vi "Сканер.vi"() -> ()   [LabVIEW 2016]
uses:
  <vilib>/Instr/_visa.llb/VISA Open Access Mode.ctl
  <vilib>/Instr/_visa.llb/VISA Configure Serial Port (Instr).vi
panel:
  out "duplicate session (F)":bool
  out "read buffer":string
  out "Gauge":dbl(knob)
  out "ScrollPosBool":bool
  out "Serial Settings:Number of Bytes at Serial Port":u32
  in  "XON/XOFF Символ":cluster{"XON":u8, "XOFF":u8}={"XON"=17, "XOFF"=19} {"XOFF" items=["NUL", "SOH", "STX", "ETX", "EOT", "ENQ", "ACK", "BEL", "BS", "HT", "LF", "VT", "FF", "CR", "SO", "SI", "DLE", "DC1", "DC2", "DC3", "DC4", "NAK", "SYN", "ETB", "CAN", "EM", "SUB", "ESC", "FS", "GS", "RS", "US", "SP", "!", "\"", "#", "$", "%", "&", "'", "(", ")", "*", "+", ",", "- (-)", ".", "/", "0", "1", "2", "3", "4", "5", "6", "7", "8", "9", ":", ";", "<", "=", ">", "?", "@", "A", "B", "C", "D", "E", "F", "G", "H", "I", "J", "K", "L", "M", "N", "O", "P", "Q", "R", "S", "T", "U", "V", "W", "X", "Y", "Z", "[", "\\", "]", "^", "_", "`", "a", "b", "c", "d", "e", "f", "g", "h", "i", "j", "k", "l", "m", "n", "o", "p", "q", "r", "s", "t", "u", "v", "w", "x", "y", "z", "{", "|", "}", "~"]; "XON" items=["NUL", "SOH", "STX", "ETX", "EOT", "ENQ", "ACK", "BEL", "BS", "HT", "LF", "VT", "FF", "CR", "SO", "SI", "DLE", "DC1", "DC2", "DC3", "DC4", "NAK", "SYN", "ETB", "CAN", "EM", "SUB", "ESC", "FS", "GS", "RS", "US", "SP", "!", "\"", "#", "$", "%", "&", "'", "(", ")", "*", "+", ",", "- (-)", ".", "/", "0", "1", "2", "3", "4", "5", "6", "7", "8", "9", ":", ";", "<", "=", ">", "?", "@", "A", "B", "C", "D", "E", "F", "G", "H", "I", "J", "K", "L", "M", "N", "O", "P", "Q", "R", "S", "T", "U", "V", "W", "X", "Y", "Z", "[", "\\", "]", "^", "_", "`", "a", "b", "c", "d", "e", "f", "g", "h", "i", "j", "k", "l", "m", "n", "o", "p", "q", "r", "s", "t", "u", "v", "w", "x", "y", "z", "{", "|", "}", "~"]}
  in  "Ошибка порта":T1
  in  "Номер COM порта":refnum<visa-resource-name>
  in  "Clear":bool
  in  "ReadStringON":bool
  in  "WriteStringON":bool
  in  "В конце записи добавить идентификатор завершения":bool=TRUE
  out "IndStartStop":bool
  in  "Exit":bool
  in  "Start":bool
  in  "Stop":bool
  out "Return Count Read":u32
  in  "В конце чтения добавить идентификатор завершения":bool=TRUE
  in  "Идентификатор завершения":u8=10 format="%.0x"
  out "Read String":string
  out "Return Count Write":u32
  in  "Write String":string="*IDN?"
  in  "Параметры порта":T2={"Бит в секунду: "=9600, "Биты данных:"=8, "Чётность"=0, "Стоповые биты"=10, "Управление потоком"=0} {"Управление потоком" items=["Нет"=0, "Xon/Xoff"=1, "RTS/CTS"=2, "DTR/DSR"=4]; "Стоповые биты" items=["1.0"=10, "1.5"=15, "2.0"=20]; "Чётность" items=["Нет", "Нечётный", "Чётный", "Маркер", "Пробел"]; "Биты данных:" items=["4"=4, "5"=5, "6"=6, "7"=7, "8"=8]; "Бит в секунду:" items=["75"=75, "110"=110, "134"=134, "150"=150, "300"=300, "600"=600, "1200"=1200, "1800"=1800, "2400"=2400, "4800"=4800, "7200"=7200, "9600"=9600, "14400"=14400, "19200"=19200, "28800"=28800, "38400"=38400, "56000"=56000, "57600"=57600, "115200"=115200, "128000"=128000, "230400"=230400]}
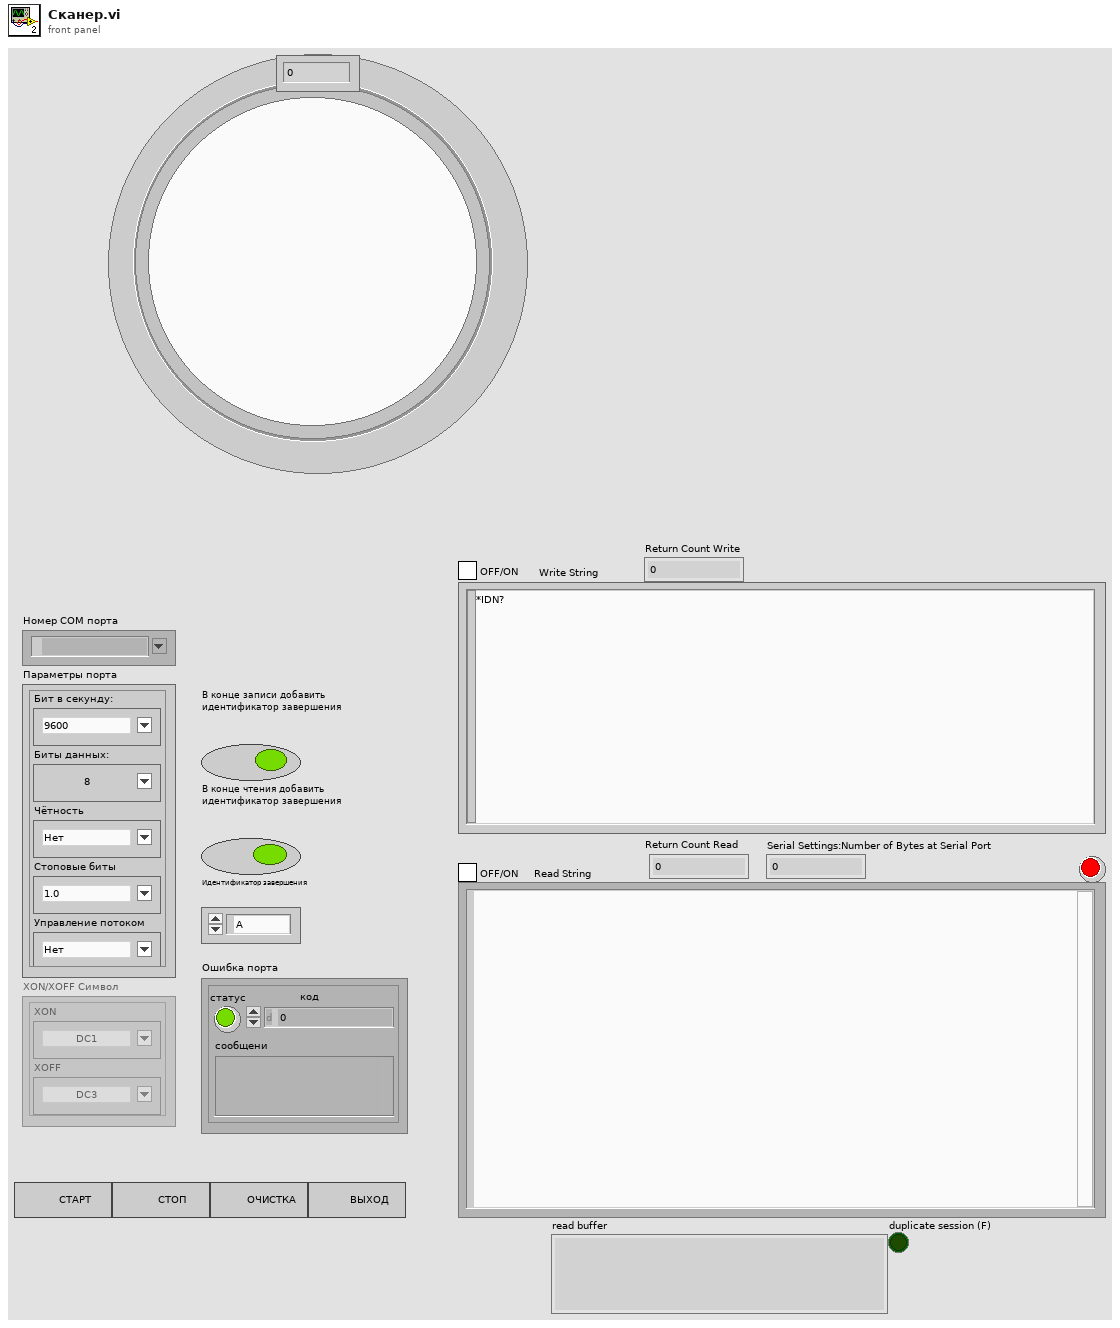
[diagram p1: front panel]
types:
  T1 = cluster{"статус":bool, "код":i32, "сообщени":string}
  T2 = cluster{"Бит в секунду: ":u32, "Биты данных:":u16, "Чётность":u16, "Стоповые биты":u16, "Управление потоком":u16}
  T3 = enum8{"Enabled", "Disabled", "Disabled and Grayed Out"}
  T4 = typedef "VISA Open Access Mode.ctl" = u32
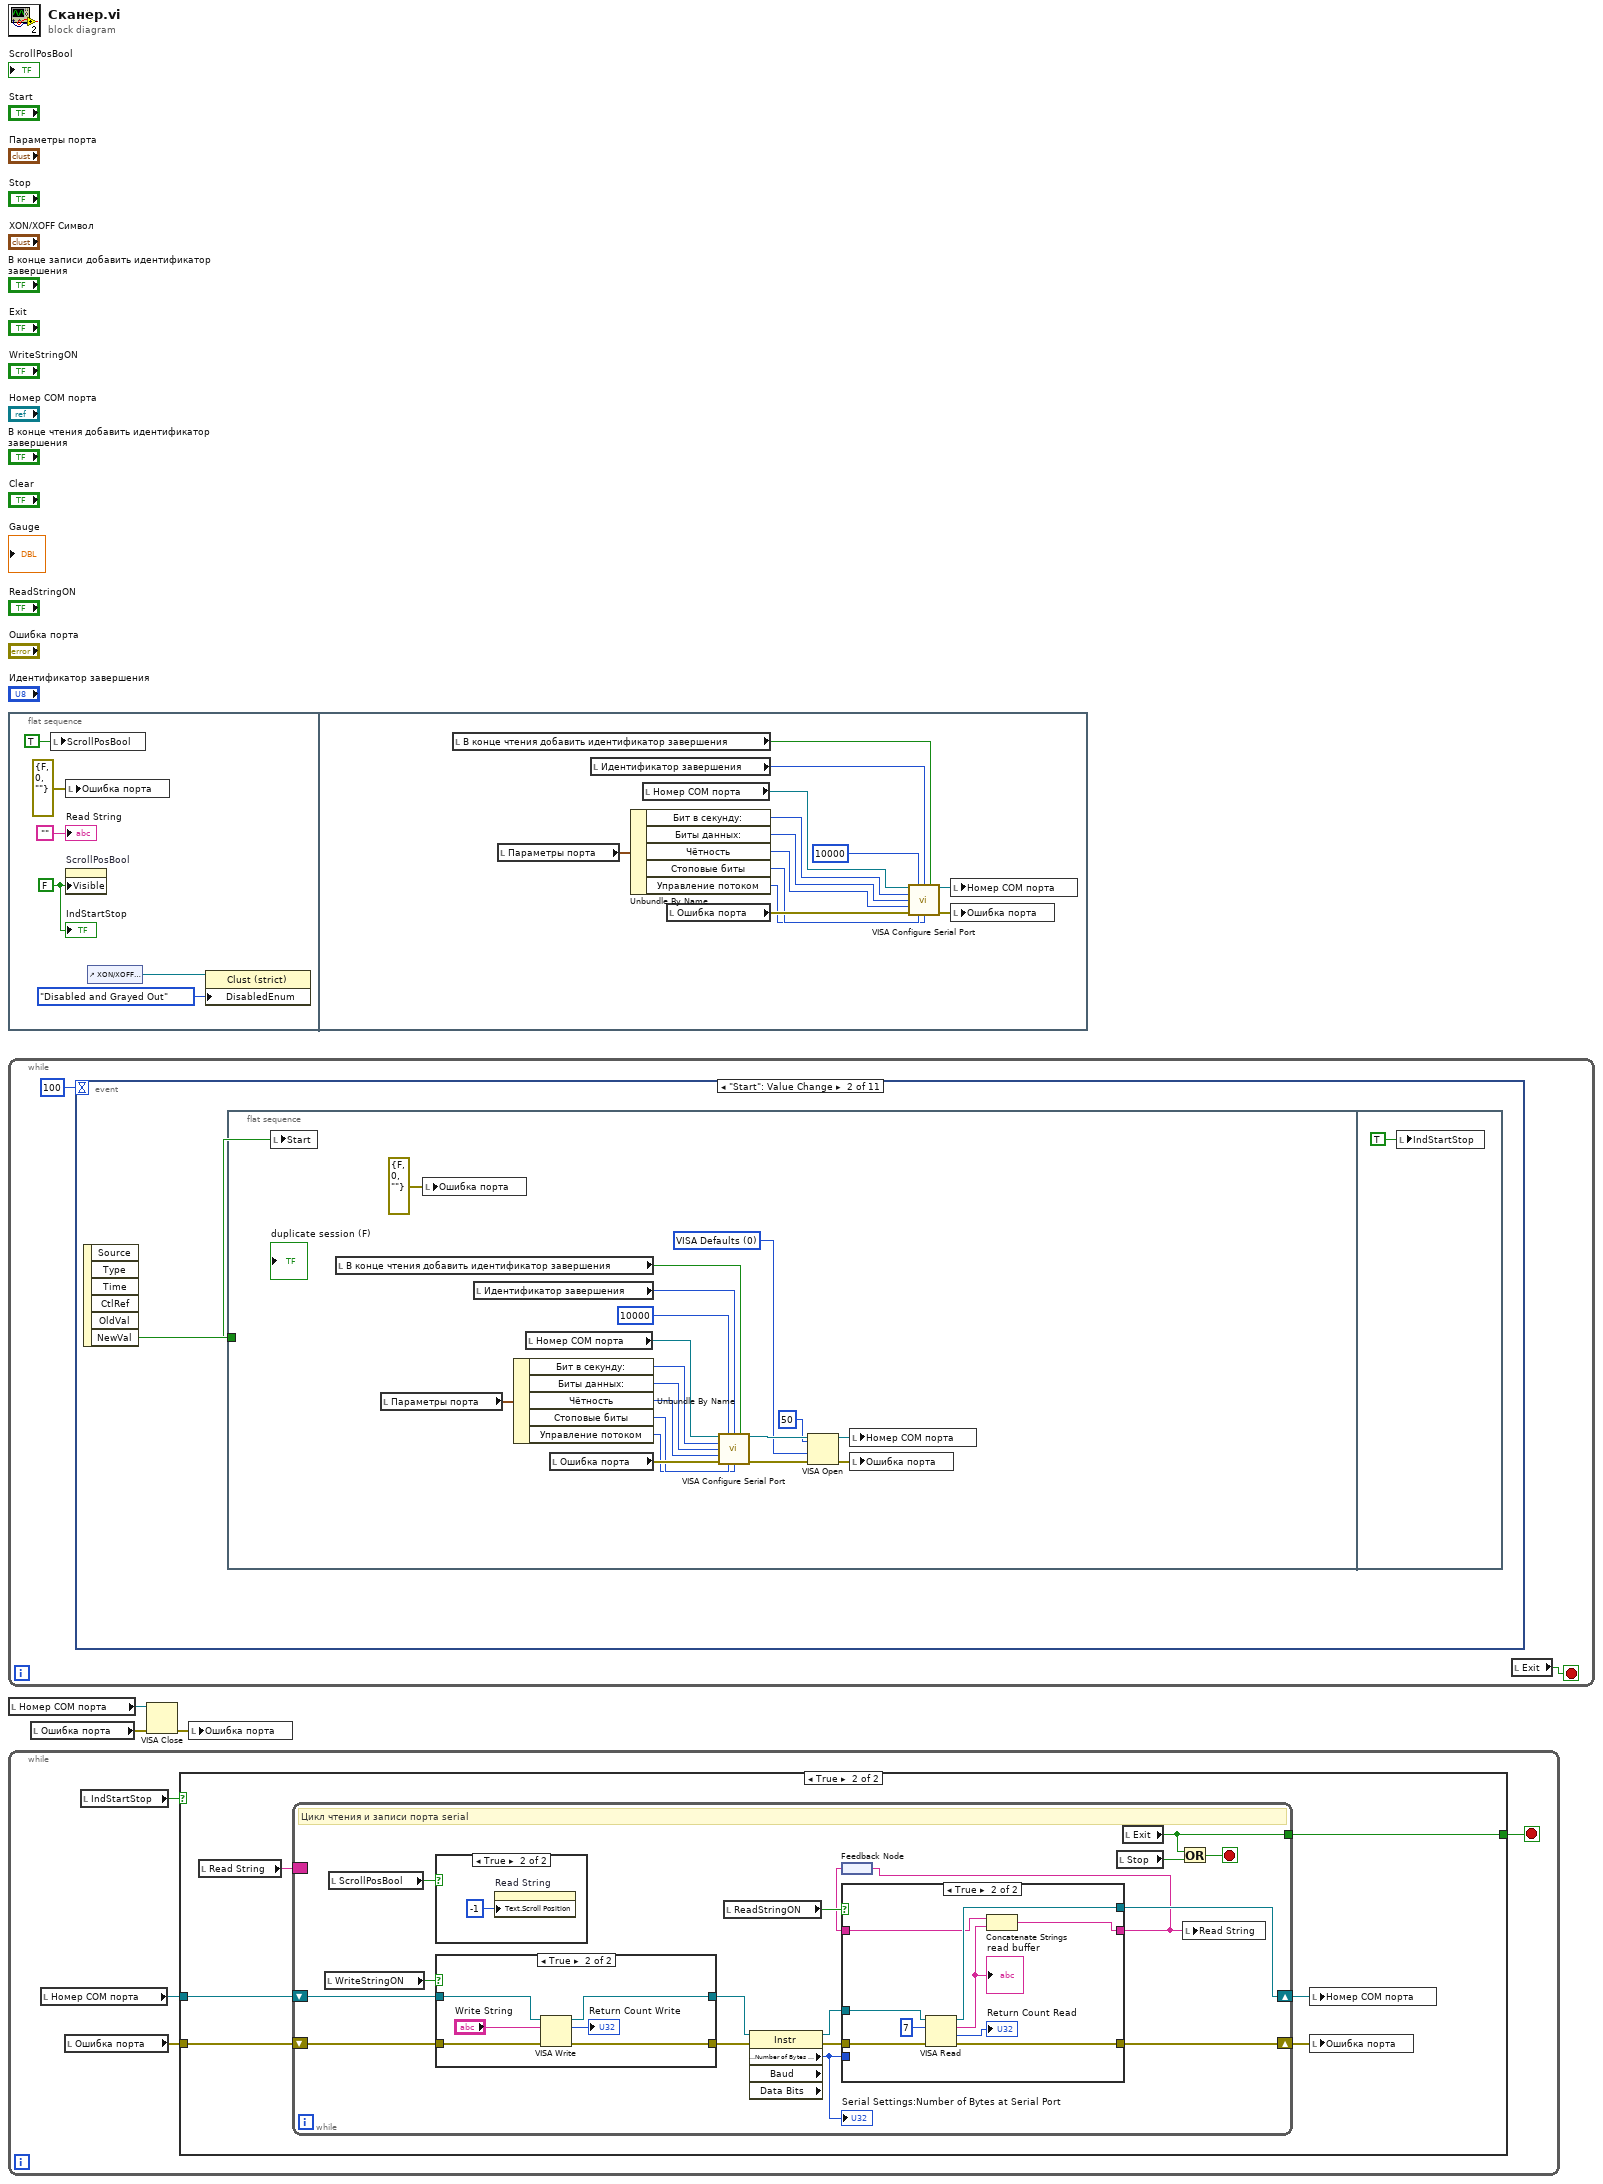
[diagram p0: block diagram]
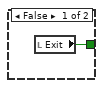
[diagram p2: hidden frame]
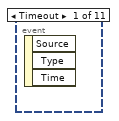
[diagram p6: hidden frame]
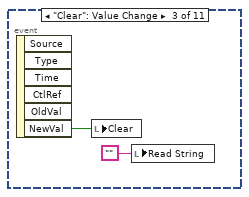
[diagram p7: hidden frame]
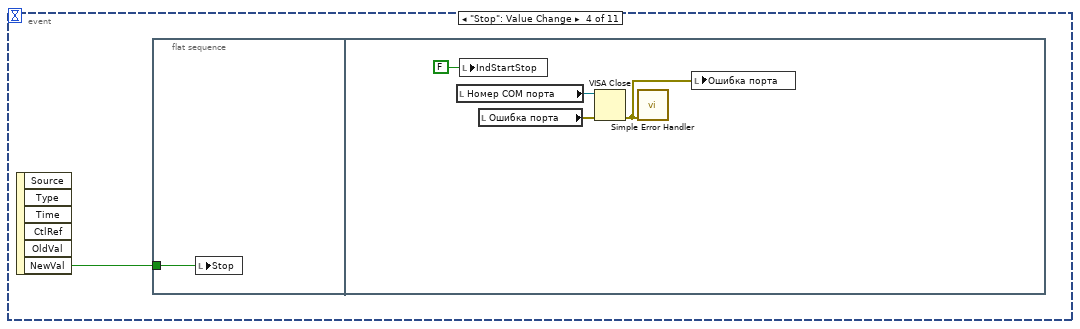
[diagram p8: hidden frame]
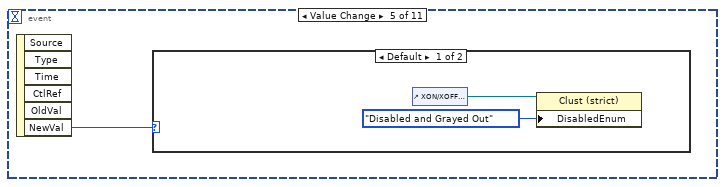
[diagram p9: hidden frame]
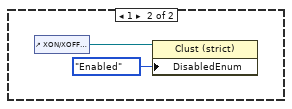
[diagram p10: hidden frame]
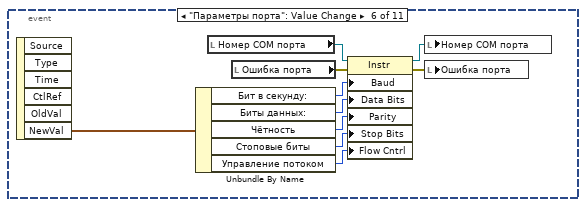
[diagram p11: hidden frame]
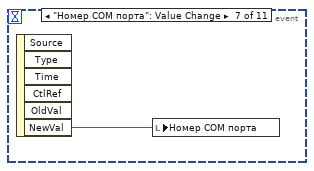
[diagram p12: hidden frame]
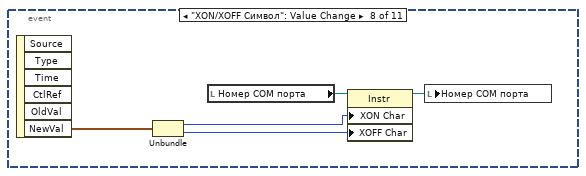
[diagram p13: hidden frame]
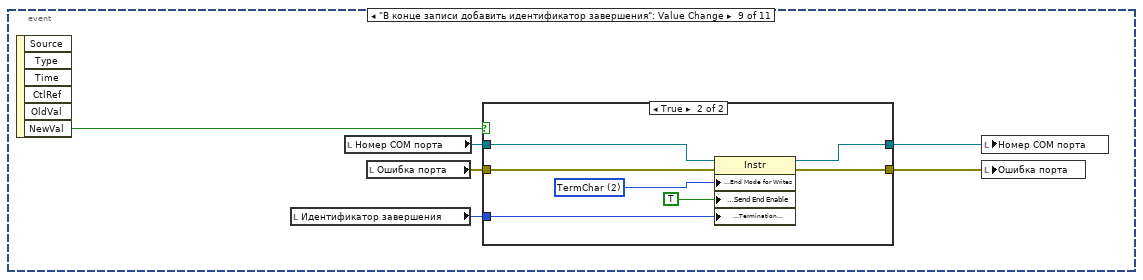
[diagram p14: hidden frame]
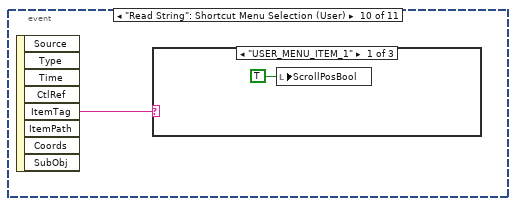
[diagram p16: hidden frame]
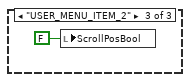
[diagram p18: hidden frame]
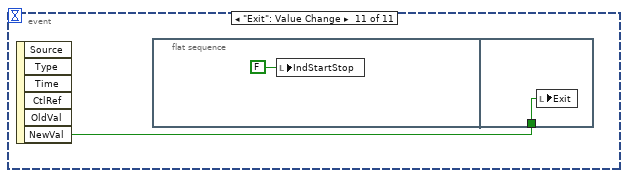
[diagram p19: hidden frame]
diagram:
  n1 = flat-sequence {
    frame #0 {
      w4 = FALSE
      n2 = local write "ScrollPosBool"(TRUE ("ScrollPosBool")) -> ()
      n3 = local write "Ошибка порта"(errorcluster {"status"=FALSE, "code"=0, "source"=""} ("error in (no error)")) -> ()
      n4 = property on="ScrollPosBool" class="Bool (strict)"("Visible"=w4) -> ()  [unwired: 2 in, 2 out]
      n5 = control-ref of="XON/XOFF Символ"() -> (w8:refnum<vi>)
      n6 = property class="Clust (strict)"(reference=w8, "DisabledEnum"=T3."Disabled and Grayed Out" ("Disabled")) -> ()  [unwired: 1 in, 2 out]
      "IndStartStop" <- w4
      "Read String" <- ""
    }
    frame #1 {
      n7 = local read "В конце чтения добавить идентификатор завершения"() -> (w21:bool)
      n8 = local read "Параметры порта"() -> (w17:T2)
      n9 = local read "Идентификатор завершения"() -> (w20:u8)
      n10 = Unbundle By Name(w17) -> ("Бит в секунду:"=w16:u32, "Биты данных:"=w15:u16, "Чётность"=w14:u16, "Стоповые биты"=w13:u16, "Управление потоком"=w12:u16)
      n11 = local read "Номер COM порта"() -> (w18:refnum<visa-resource-name>)
      n12 = local read "Ошибка порта"() -> (w19:T1)
      n13 = call-poly "VISA Configure Serial Port"("VISA resource name"=w18, "timeout (10sec)"=u32 10000, "termination char\n(0xA = '\\n' = LF)"=w20, "Enable Termination\nChar (T)"=w21, "baud rate (9600)"=w16, "data bits (8)"=w15, "parity (0:none)"=w14, "error in (no error)"=w19, "stop bits (10: 1 bit)"=w13, "flow control (0:none)"=w12) -> ("VISA resource name out"=w11:refnum<visa-resource-name>, "error out"=w10:errorcluster)  [unwired: 4 in]
      n14 = local write "Номер COM порта"(w11) -> ()
      n15 = local write "Ошибка порта"(w10) -> ()
    }
  }
  n16 = while {
    stop <- w23 stop-if-true
    n17 = event shown="[1] \"Start\": Value Change" {
      selector: _ -> [_ _ _ _ _ _ _ _ _ _ _]
      dyn-events: _ -> [_ _ _ _ _ _ _ _ _ _ _]
      timeout: 100 -> [_ _ _ _ _ _ _ _ _ _ _]
      event Timeout {
        n18 = event-data() -> ()  [unwired: 1 in, 3 out]
      }
      event "Start": Value Change {
        n19 = event-data() -> ("NewVal"=w25:bool)  [unwired: 1 in, 5 out]
        n20 = flat-sequence {
          tunnel: w25 -> [w44]
          frame #0 {
            w26 = T4 0 items=["VISA Defaults"=0, "Exclusive Lock"=1, "Load Configured Settings"=4] ("Access Mode")
            n21 = local write "Start"(w44) -> ()
            n22 = local read "В конце чтения добавить идентификатор завершения"() -> (w41:bool)
            n23 = local read "Параметры порта"() -> (w37:T2)
            n24 = local write "Ошибка порта"(errorcluster {"status"=FALSE, "code"=0, "source"=""} ("error in (no error)")) -> ()
            n25 = local read "Идентификатор завершения"() -> (w40:u8)
            n26 = Unbundle By Name(w37) -> ("Бит в секунду:"=w36:u32, "Биты данных:"=w35:u16, "Чётность"=w34:u16, "Стоповые биты"=w33:u16, "Управление потоком"=w32:u16)
            n27 = local read "Номер COM порта"() -> (w38:refnum<visa-resource-name>)
            n28 = local read "Ошибка порта"() -> (w39:T1)
            n29 = call-poly "VISA Configure Serial Port"("VISA resource name"=w38, "timeout (10sec)"=u32 10000, "termination char\n(0xA = '\\n' = LF)"=w40, "Enable Termination\nChar (T)"=w41, "baud rate (9600)"=w36, "data bits (8)"=w35, "parity (0:none)"=w34, "error in (no error)"=w39, "stop bits (10: 1 bit)"=w33, "flow control (0:none)"=w32) -> ("VISA resource name out"=w31:refnum<visa-resource-name>, "error out"=w30:errorcluster)  [unwired: 4 in]
            n30 = VISA Open(timeout (0)=u32 50 ("VISA Open timeout (0)"), access mode=w26, error in (no error)=w30, VISA resource name=w31) -> (VISA resource name=w28:refnum<visa-resource-name>, error out=w27:errorcluster)  [unwired: 1 in]
            n31 = local write "Номер COM порта"(w28) -> ()
            n32 = local write "Ошибка порта"(w27) -> ()
          }
          frame #1 {
            n33 = local write "IndStartStop"(TRUE) -> ()
          }
        }
      }
      event "Clear": Value Change {
        n34 = event-data() -> ("NewVal"=w47:bool)  [unwired: 1 in, 5 out]
        n35 = local write "Clear"(w47) -> ()
        n36 = local write "Read String"("") -> ()
      }
      event "Stop": Value Change {
        n37 = event-data() -> ("NewVal"=w48:bool)  [unwired: 1 in, 5 out]
        n38 = flat-sequence {
          tunnel: w48 -> [w49]
          frame #0 {
            n39 = local write "Stop"(w49) -> ()
          }
          frame #1 {
            n40 = local read "Номер COM порта"() -> (w51:refnum<visa-resource-name>)
            n41 = local write "IndStartStop"(FALSE) -> ()
            n42 = local read "Ошибка порта"() -> (w50:T1)
            n43 = VISA Close(VISA resource name=w51, error in (no error)=w50) -> (error out=w52:errorcluster)
            n44 = call <vilib>:"Simple Error Handler.vi"("error in (no error)"=w52) -> ()  [unwired: 1 in, 8 out]
            n45 = local write "Ошибка порта"(w52) -> ()
          }
        }
      }
      event "Параметры порта.Управление потоком": Value Change {
        n46 = event-data() -> ("NewVal"=w54:u16)  [unwired: 1 in, 5 out]
        n47 = case shown="Default" w54 {
          frame Default {
            n48 = control-ref of="XON/XOFF Символ"() -> (w55:refnum<vi>)
            n49 = property class="Clust (strict)"(reference=w55, "DisabledEnum"=T3."Disabled and Grayed Out" ("Disabled")) -> ()  [unwired: 1 in, 2 out]
          }
          frame 1 {
            n50 = control-ref of="XON/XOFF Символ"() -> (w57:refnum<vi>)
            n51 = property class="Clust (strict)"(reference=w57, "DisabledEnum"=T3."Enabled" ("Disabled")) -> ()  [unwired: 1 in, 2 out]
          }
        }
      }
      event "Параметры порта": Value Change {
        n52 = event-data() -> ("NewVal"=w68:T2)  [unwired: 1 in, 5 out]
        n53 = Unbundle By Name(w68) -> ("Бит в секунду:"=w63:u32, "Биты данных:"=w62:u16, "Чётность"=w61:u16, "Стоповые биты"=w60:u16, "Управление потоком"=w59:u16)
        n54 = local read "Номер COM порта"() -> (w67:refnum<visa-resource-name>)
        n55 = local read "Ошибка порта"() -> (w66:T1)
        n56 = property class="Instr"(reference=w67, error in=w66, "Baud"=w63, "Data Bits"=w62, "Parity"=w61, "Stop Bits"=w60, "Flow Cntrl"=w59) -> (reference out=w65:refnum<visa-resource-name>, error out=w64:errorcluster)
        n57 = local write "Номер COM порта"(w65) -> ()
        n58 = local write "Ошибка порта"(w64) -> ()
      }
      event "Номер COM порта": Value Change {
        n59 = event-data() -> ("NewVal"=w69:refnum<visa-resource-name>)  [unwired: 1 in, 5 out]
        n60 = local write "Номер COM порта"(w69) -> ()
      }
      event "XON/XOFF Символ": Value Change {
        n61 = event-data() -> ("NewVal"=w72:cluster{"XON":u8, "XOFF":u8})  [unwired: 1 in, 5 out]
        n62 = Unbundle(w72) -> ("XON"=w71:u8, "XOFF"=w70:u8)
        n63 = local read "Номер COM порта"() -> (w74:refnum<visa-resource-name>)
        n64 = property class="Instr"(reference=w74, "XON Char"=w71, "XOFF Char"=w70) -> (reference out=w73:refnum<visa-resource-name>)  [unwired: 1 in, 1 out]
        n65 = local write "Номер COM порта"(w73) -> ()
      }
      event "В конце записи добавить идентификатор завершения": Value Change {
        n66 = event-data() -> ("NewVal"=w79:bool)  [unwired: 1 in, 5 out]
        n67 = local read "Идентификатор завершения"() -> (w80:u8)
        n68 = local read "Номер COM порта"() -> (w78:refnum<visa-resource-name>)
        n69 = local read "Ошибка порта"() -> (w76:T1)
        n70 = case shown="True" w79 {
          tunnel: w80 -> [_ w85]
          tunnel: w78 -> [_ w84]
          tunnel: [_ w83] -> w77
          tunnel: w76 -> [_ w82]
          tunnel: [_ w81] -> w75
          frame False {
          }
          frame True {
            w87 = u16 2 items=["None", "LastBit", "TermChar", "Break"] ("Serial Settings:Serial End Mode for Writes")
            n71 = property class="Instr"(reference=w84, error in=w82, "Serial Settings:End Mode for Writes"=w87, "Message Based Settings:Send End Enable"=TRUE, "Message Based Settings:Termination Character"=w85) -> (reference out=w83:refnum<visa-resource-name>, error out=w81:errorcluster)
          }
        }
        n72 = local write "Номер COM порта"(w77) -> ()
        n73 = local write "Ошибка порта"(w75) -> ()
      }
      event "Read String": Shortcut Menu Selection (User) {
        n74 = event-data() -> ("ItemTag"=w88:string)  [unwired: 1 in, 7 out]
        n75 = case shown="\"USER_MENU_ITEM_1\"" w88 {
          frame "USER_MENU_ITEM_1" {
            n76 = local write "ScrollPosBool"(TRUE ("ScrollPosBool")) -> ()
          }
          frame Default {
          }
          frame "USER_MENU_ITEM_2" {
            n77 = local write "ScrollPosBool"(FALSE ("ScrollPosBool")) -> ()
          }
        }
      }
      event "Exit": Value Change {
        n78 = event-data() -> ("NewVal"=w91:bool)  [unwired: 1 in, 5 out]
        n79 = flat-sequence {
          tunnel: w91 -> [w93]
          frame #0 {
            n80 = local write "IndStartStop"(FALSE) -> ()
          }
          frame #1 {
            n81 = local write "Exit"(w93) -> ()
          }
        }
      }
    }
    n82 = local read "Exit"() -> (w23:bool)
  }
  n83 = local read "Номер COM порта"() -> (w2:refnum<visa-resource-name>)
  n84 = while {
    stop <- w94 stop-if-true
    n85 = local read "Номер COM порта"() -> (w96:refnum<visa-resource-name>)
    n86 = local read "Ошибка порта"() -> (w95:T1)
    n87 = local read "IndStartStop"() -> (w97:bool)
    n88 = case shown="True" w97 {
      tunnel: w96 -> [_ w104]
      tunnel: w95 -> [_ w103]
      tunnel: [w98 w99] -> w94
      frame False {
        n89 = local read "Exit"() -> (w98:bool)
      }
      frame True {
        n90 = local read "Read String"() -> (w100:string)
        n91 = while {
          shift-right: [w110] -> w101
          shift-left: w104 -> [w119]
          shift-right: [w109] -> w102
          shift-left: w103 -> [w118]
          border: w100 -> [_]
          tunnel: [w106] -> w99
          stop <- w113 stop-if-true
          # "Цикл чтения и записи порта serial"
          n92 = local read "WriteStringON"() -> (w115:bool)
          n93 = local read "ScrollPosBool"() -> (w107:bool)
          n94 = case shown="True" w107 {
            frame False {
            }
            frame True {
              n95 = property on="Read String" class="Str"("Text.Scroll Position"=-1) -> ()  [unwired: 2 in, 2 out]
            }
          }
          n96 = case shown="True" w115 {
            tunnel: [w136 w142] -> w121
            tunnel: [w135 w141] -> w120
            tunnel: w119 -> [w136 w140]
            tunnel: w118 -> [w135 w139]
            frame False {
            }
            frame True {
              n97 = VISA Write(VISA resource name=w140, write buffer="Write String", error in (no error)=w139) -> (VISA resource name out=w142:refnum<visa-resource-name>, return count=→"Return Count Write":u32, error out=w141:errorcluster)
            }
          }
          n98 = local read "ReadStringON"() -> (w114:bool)
          n99 = property class="Instr" props=["Serial Settings:Number of Bytes at Serial Port", "Baud", "Data Bits"](reference=w121, error in=w120) -> (reference out=w117:refnum<visa-resource-name>, error out=w116:errorcluster, "Serial Settings:Number of Bytes at Serial Port"=w111:u32)  [unwired: 2 out]
          "Serial Settings:Number of Bytes at Serial Port" <- w111
          n100 = feedback #1() -> (w108:string)
          n101 = case shown="True" w114 {
            tunnel: [w125 w134] -> w110
            tunnel: [w124 w130] -> w109
            tunnel: w111 -> [_ _]
            tunnel: w117 -> [w125 w133]
            tunnel: w116 -> [w124 w132]
            tunnel: w108 -> [w123 w128]
            tunnel: [w123 w129] -> w105
            frame False {
            }
            frame True {
              n102 = VISA Read(VISA resource name=w133, byte count=u32 7, error in (no error)=w132) -> (VISA resource name out=w134:refnum<visa-resource-name>, read buffer=w127:string, return count=→"Return Count Read":u32, error out=w130:errorcluster)
              "read buffer" <- w127
              n103 = Concatenate Strings(w128, w127) -> (w129:string)
            }
          }
          n104 = feedback-in #1(w105) -> ()
          n105 = local read "Stop"() -> (w112:bool)
          n106 = local read "Exit"() -> (w106:bool)
          n107 = Or(x=w106, y=w112) -> (x .or. y?=w113:bool)
          n108 = local write "Read String"(w105) -> ()
        }
        n109 = local write "Номер COM порта"(w101) -> ()
        n110 = local write "Ошибка порта"(w102) -> ()
      }
    }
  }
  n111 = local read "Ошибка порта"() -> (w3:T1)
  n112 = VISA Close(VISA resource name=w2, error in (no error)=w3) -> (error out=w1:errorcluster)
  n113 = local write "Ошибка порта"(w1) -> ()
